vi "virtual Z for virtual joystick jog.vi"(11 "virtual Z relative":dbl) -> (3 "virtual motion string":string)   [LabVIEW 2012]
doc: "SciScan 1.2 160622"
uses:
  GFG/GFGnumericGet.vi
  GFG/GFGbooleanGet.vi
  GFG/GFG library.lvlib
panel:
  in  "y":dbl=10.0
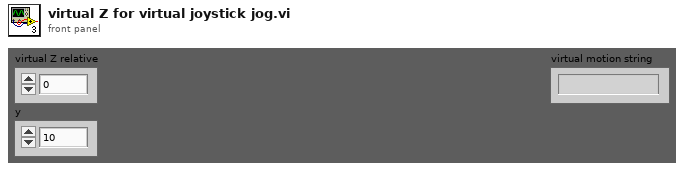
[diagram p1: front panel]
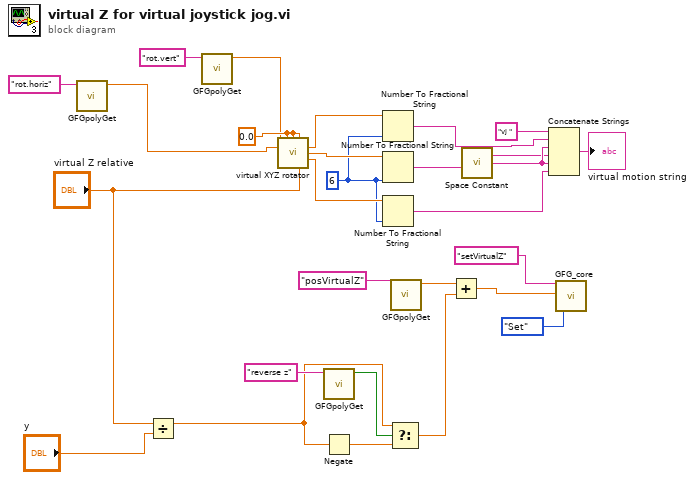
[diagram p0: block diagram]
diagram:
  w13 = i16 6 ("precision (6)")
  w22 = 0.0 ("current pos X")
  n1 = call-poly "GFGpolyGet.vi"("Variable Name in"="rot.horiz") -> ("Numeric"=w21:dbl)  [unwired: 8 in, 2 out]
  n2 = Divide(x="virtual Z relative", y="y") -> (x/y=w7:dbl)
  n3 = call-poly "GFGpolyGet.vi"("Variable Name in"="rot.vert") -> ("Numeric"=w20:dbl)  [unwired: 8 in, 2 out]
  n4 = call "virtual XYZ rotator.vi"("vertical (cw is pos)"=w20, "current pos X"=w22, "current pos Y"=w22, "current pos Z"=w22, "horizontal (cw is pos)"=w21, "virtual Z relative"="virtual Z relative") -> ("new pos X"=w25:dbl, "new pos Y"=w26:dbl, "new pos Z"=w27:dbl)  [unwired: 7 in]
  n5 = call-poly "GFGpolyGet.vi"("Variable Name in"="reverse z") -> ("Boolean Value OUT"=w11:bool)  [unwired: 9 in, 1 out]
  n6 = Negate(x=w7) -> (-x=w10:dbl)
  n7 = Number To Fractional String(number=w25, precision (6)=w13) -> (F-format string=w18:string)  [unwired: 2 in]
  n8 = Number To Fractional String(number=w26, precision (6)=w13) -> (F-format string=w16:string)  [unwired: 2 in]
  n9 = Number To Fractional String(number=w27, precision (6)=w13) -> (F-format string=w15:string)  [unwired: 2 in]
  n10 = Select(t=w7, s=w11, f=w10) -> (s? t:f=w12:dbl)
  n11 = call-poly "GFGpolyGet.vi"("Variable Name in"="posVirtualZ") -> ("Numeric"=w3:dbl)  [unwired: 8 in, 2 out]
  n12 = Add(x=w3, y=w12) -> (x+y=w4:dbl)
  n13 = call <vilib>:"Space Constant.vi"() -> ("String"=w17:string)
  n14 = Concatenate Strings("vj " ("string"), w18, w17, w16, w17, w15) -> (→"virtual motion string":string)
  n15 = call "GFG_core.vi"("Variable Name in"="setVirtualZ", "Variant in"=w4, "Action"=enum16{"Init", "Set", "Get"}."Set") -> ()  [unwired: 10 in, 7 out]
